vi "Lookup Manager by Path.vi"(8 "error in (no error)":errorcluster, 10 "Path":string, 11 "WebSocket Handler in":refnum<class "WebSocket Handler.lvclass">) -> (0 "error out":errorcluster, 2 "Manager":refnum<class "WebSocket Manager.lvclass">, 3 "WebSocket Handler out":refnum<class "WebSocket Handler.lvclass">)   [LabVIEW 2020, in "HTTP Server.lvlib" / "WebSocket Handler.lvclass"]
uses:
  WebSocket Handler.lvclass
  WebSocket Handler.lvclass/WebSocket Handler.ctl
  WebSocket Manager/WebSocket Manager.lvclass
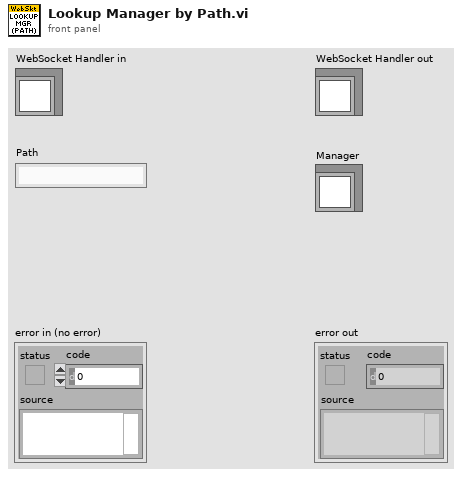
[diagram p1: front panel]
types:
  T1 = typedef "HTTP Server.lvlib/WebSocket Data.ctl" = cluster{"WS Managers":map{string, refnum<class "WebSocket Manager.lvclass">}}
  T2 = map{string, refnum<class "WebSocket Manager.lvclass">}
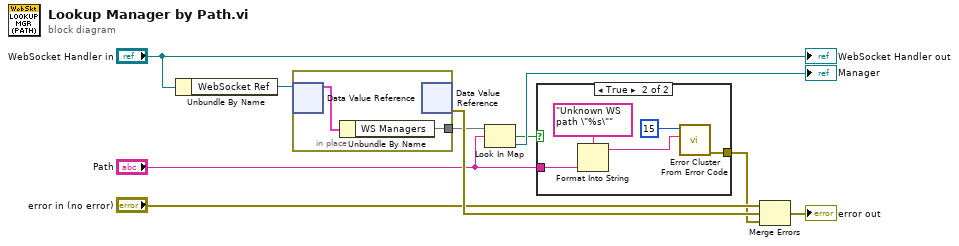
[diagram p0: block diagram]
diagram:
  n1 = Unbundle By Name("WebSocket Handler in") -> ("WebSocket Ref"=w8:refnum<data-value>)
  n2 = in-place {
    in-place-border: [w11] -> w7
    n3 = in-place-dvr #1(w8) -> (w12:T1)  [unwired: 1 out]
    n4 = Unbundle By Name(w12) -> ("WS Managers"=w11:T2)
    n5 = in-place-dvr #1() -> (w10:errorcluster)  [unwired: 1 in, 1 out]
  }
  n6 = Look In Map(map=w7, key="Path") -> (key not found?=w3:bool, value=→"Manager":refnum<class "WebSocket Manager.lvclass">)  [unwired: 1 in]
  n7 = case shown="True" w3 {
    tunnel: "Path" -> [_ w15]
    tunnel: [_ w17] -> w1
    frame False {
    }
    frame True {
      n8 = Format Into String(format string="Unknown WS path \"%s\"", w15) -> (resulting string=w13:string)  [unwired: 2 in, 1 out]
      n9 = call <vilib>:"Error Cluster From Error Code.vi"("error message (\"\")"=w13, "error code (0)"=15) -> ("error out"=w17:errorcluster)  [unwired: 7 in]
    }
  }
  n10 = Merge Errors("error in (no error)", w10, w1) -> (→"error out":errorcluster)
  "WebSocket Handler out" <- "WebSocket Handler in"
